vi "Leap Motion testing.vi"() -> ()   [LabVIEW 2014]
uses:
  <vilib>/MakerHub/Leap/Public/Instance VIs/Read N Point Positions Velocities.vi
  <vilib>/MakerHub/Leap/Public/Instance VIs/Read N Hand Positions Velocities.vi
  <vilib>/MakerHub/Leap/LMH-Leap.lvlib
panel:
  out "fingers":i32
  out "Hand Positions":cluster{"X":sgl, "Y":sgl, "Z":sgl}[](array[cluster])
  out "Point Positions":cluster{"X":sgl, "Y":sgl, "Z":sgl}[](array[cluster])
  in  "stop":bool
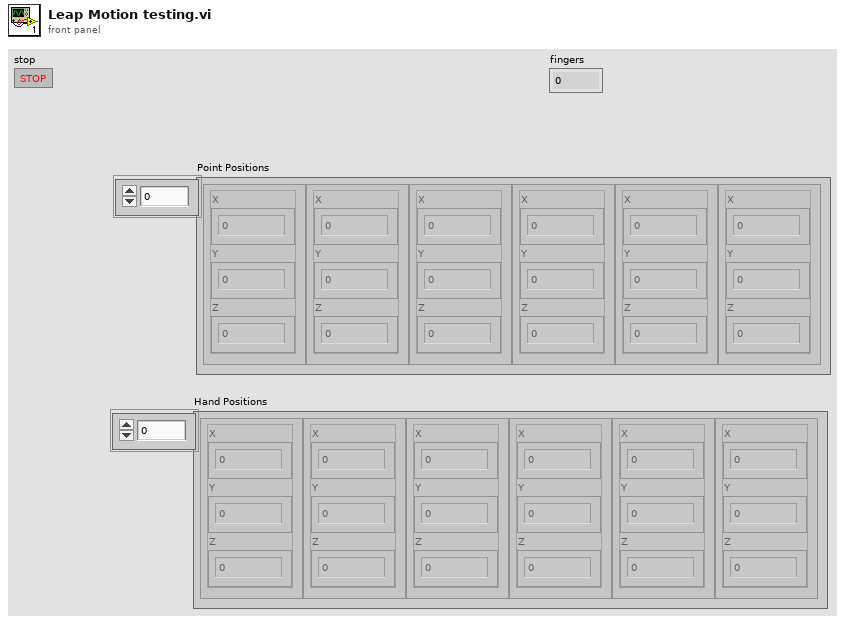
[diagram p1: front panel]
types:
  T1 = typedef "LMH-Leap.lvlib/Leap Handle.ctl" = cluster{"LeapCSharp":refnum<k24>}
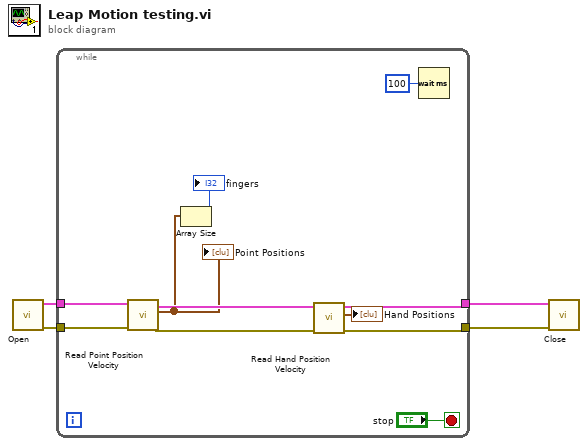
[diagram p0: block diagram]
diagram:
  n1 = call <vilib>:"Open.vi"() -> ("Error Out"=w4:errorcluster, "Leap Handle"=w3:T1)  [unwired: 10 in]
  n2 = while {
    tunnel: w4 -> [w13]
    tunnel: w3 -> [w12]
    tunnel: [w9] -> w2
    tunnel: [w8] -> w1
    stop <- "stop" stop-if-true
    n3 = call-poly <vilib>:"Read Point Position Velocity.vi"("Error In"=w13, "Leap Handle"=w12) -> ("Error Out"=w11:errorcluster, "Point Positions"=w6:cluster{"X":sgl, "Y":sgl, "Z":sgl}[], "Leap Handle"=w10:T1)  [unwired: 6 in, 1 out]
    "Point Positions" <- w6
    n4 = Array Size(array=w6) -> (size(s)=→"fingers":i32)
    n5 = call-poly <vilib>:"Read Hand Position Velocity.vi"("Error In"=w11, "Leap Handle"=w10) -> ("Error Out"=w8:errorcluster, "Hand Positions"=→"Hand Positions":cluster{"X":sgl, "Y":sgl, "Z":sgl}[], "Leap Handle"=w9:T1)  [unwired: 6 in, 1 out]
    n6 = Wait (ms)(milliseconds to wait=u32 100) -> ()  [unwired: 1 out]
  }
  n7 = call <vilib>:"Close.vi"("Error In"=w1, "Leap Handle"=w2) -> ()  [unwired: 9 in, 1 out]
